vi "Unregister Self.vi"(11 "Self":refnum<class "UniqueName.lvclass">) -> ()   [LabVIEW 2014, in "ConfigurableQMH.lvlib"]
uses:
  ConfigurableQMH.lvlib
  <vilib>/LabVIEW Open Source Project/Unicity/UniqueName/UniqueNameClass/UniqueName.lvclass
  <vilib>/LabVIEW Open Source Project/Unicity/UniqueName/Registry/NameRegistry.lvclass
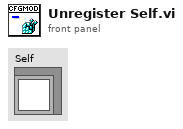
[diagram p1: front panel]
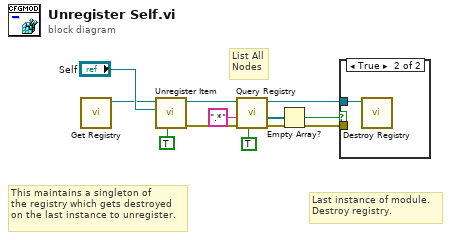
[diagram p0: block diagram]
diagram:
  # "Last instance of module.\nDestroy registry."
  # "This maintains a singleton of\nthe registry which gets destroyed\non the last instance to unregister."
  # "List All\nNodes"
  n1 = call "Get Registry.vi"() -> ("Registry"=w2:refnum<data-value>)  [unwired: 11 in]
  n2 = call <vilib>:"Unregister Item.vi"("Remove Dependencies?"=TRUE, "Node"="Self", "Registry in"=w2) -> ("error out"=w8:errorcluster, "Registry"=w7:refnum<data-value>)  [unwired: 5 in, 2 out]
  n3 = call <vilib>:"Query Registry.vi"("use Regex? (F)"=TRUE, "error in (no error)"=w8, "Search string"=".*", "Registry in"=w7) -> ("error out"=w1:errorcluster, "Nodes"=w9:refnum<class "UniqueName.lvclass">[], "Registry"=w11:refnum<data-value>)  [unwired: 3 in, 2 out]
  n4 = Empty Array?(array=w9) -> (empty?=w10:bool)
  n5 = case shown="True" w10 {
    tunnel: w11 -> [_ w12]
    tunnel: w1 -> [_ _]
    frame False {
    }
    frame True {
      n6 = call <vilib>:"Destroy Registry.vi"("Registry in"=w12) -> ()  [unwired: 9 in, 2 out]
    }
  }
